vi "Status Preset.vi"(0 "VISA resource name":refnum<visa-resource-name>, 11 "error in (no error)":errorcluster) -> (4 "VISA resource name out":refnum<visa-resource-name>, 15 "error out":errorcluster)   [LabVIEW 2020, in "NH Research Regenerative Test Series.lvlib"]
doc: "Sets the value of all the enable registers (operation and questionable) to 0 (ALL disabled).\n\nThis only affects the enable registers. It does not affect either the “status byte” or the “standard event status” as defined by IEEE 488.2. This does not clear any of the event registers or any item from the error/event queue. The *CLS command is used to clear all event registers and queues in the device status-reporting mechanism. For the SCPI mandatory status data structures, this command sets the enable registers to 0’s."
uses:
  NH Research Regenerative Test Series.lvlib
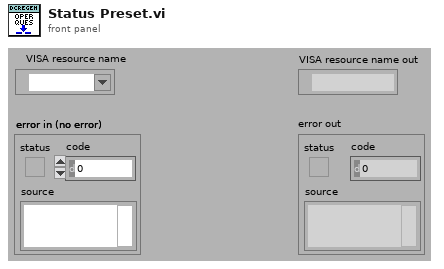
[diagram p1: front panel]
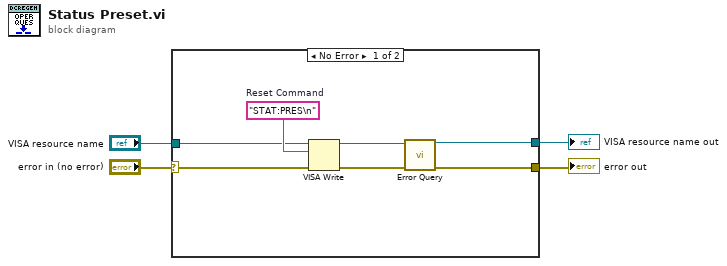
[diagram p0: block diagram]
diagram:
  n1 = case shown="No Error" "error in (no error)" {
    selector: "error in (no error)" -> [w5 w12]
    tunnel: "VISA resource name" -> [w6 w13]
    tunnel: [w11 w13] -> w3
    tunnel: [w10 w12] -> w2
    frame No Error {
      w9 = "STAT:PRES\n"  # Reset Command
      n2 = VISA Write(VISA resource name=w6, write buffer=w9, error in (no error)=w5) -> (VISA resource name out=w8:refnum<visa-resource-name>, error out=w7:errorcluster)  [unwired: 1 out]
      n3 = call "Error Query.vi"("VISA resource name"=w8, "error in (no error)"=w7) -> ("VISA resource name out"=w11:refnum<visa-resource-name>, "error out"=w10:errorcluster)  [unwired: 10 in, 2 out]
    }
    frame Error {
    }
  }
  "error out" <- w2
  "VISA resource name out" <- w3
